vi "LVClass_ModalCoef ctor from copy.vi"(0 "ModalCoef (const)":refnum<class "ModalCoef.lvclass">, 5 "ModalCoef to copy":refnum<class "ModalCoef.lvclass">, 11 "error in (no error)":errorcluster) -> (4 "ModalCoef (new)":refnum<class "ModalCoef.lvclass">, 6 "ModalCoef to copy (dup)":refnum<class "ModalCoef.lvclass">, 15 "error out":errorcluster)   [LabVIEW 2020, in "ModalCoef.lvclass"]
doc: "ModalCoef constructor.\n\n--------------------------------------------------------------------------------\n\n<B>ModalCoefIn </B> : Constant Pointer to ModalCoef object.\n<B>ModalCoefOut </B> : Constant Pointer to ModalCoef object.\n<B>TypePhase </B> : TypePhase Phase mode reconstruction.\n<B>ErrorIn </B> : Error\n<B>ErrorOut </B> : Error\n\n--------------------------------------------------------------------------------"
uses:
  ModalCoef.lvclass
  Controls/Handle creation.ctl
  ModalCoef.lvclass/ModalCoef.ctl
  LVClass_ModalCoef Read ModalCoef.vi
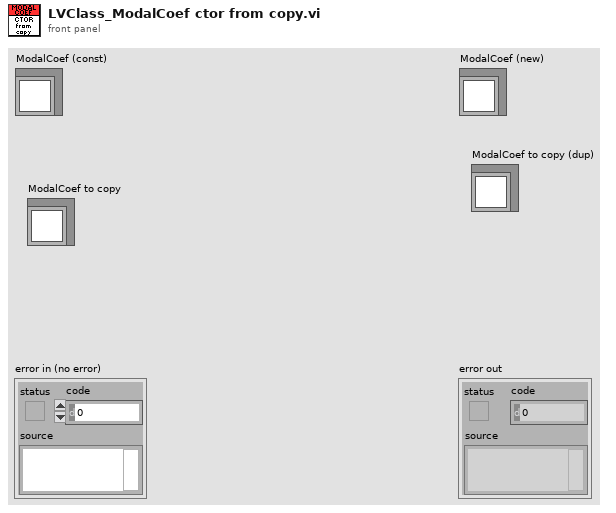
[diagram p1: front panel]
types:
  T1 = typedef "Handle creation.ctl" = enum16{"By ctor", "By write function"}
  T2 = typedef "ClassID.ctl" = i64
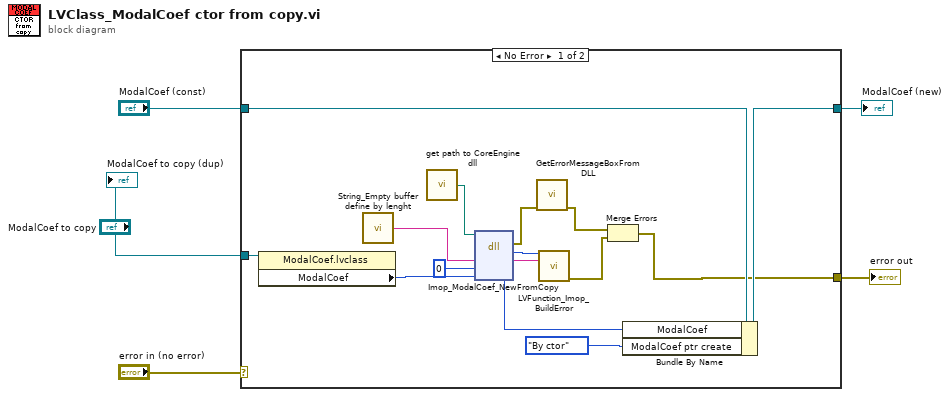
[diagram p0: block diagram]
diagram:
  n1 = case shown="No Error" "error in (no error)" {
    selector: "error in (no error)" -> [_ w22]
    tunnel: [w8 w22] -> w4
    tunnel: [w11 w21] -> w2
    tunnel: "ModalCoef (const)" -> [w12 w21]
    tunnel: "ModalCoef to copy" -> [w7 _]
    frame No Error {
      n2 = property class="ModalCoef.lvclass"(reference=w7) -> ("ModalCoef"=w6:T2)  [unwired: 1 in, 2 out]
      n3 = call "String_Empty buffer define by lenght.vi"() -> ("Empty buffer"=w20:string)  [unwired: 1 in]
      n4 = call "get path to CoreEngine dll.vi"() -> ("path to wavekit library"=w17:path)  [unwired: 14 in, 1 out]
      n5 = dll-call lib="D:/soft/HASO_v3/SVN_trunk/ImOpCoreEngine4_LV2011/DLLs/c_interface_vc100.dll" fn="Imop_ModalCoef_NewFromCopy"(path in=w17, "message"=w20, "ModalCoef"=0 ("Pupil"), "ModalCoefToCopy"=w6) -> (error out=w16:errorcluster, "return type"=w18:i32, "message"=w19:string, "ModalCoef"=w14:i64)  [unwired: 3 in, 1 out]
      n6 = call "GetErrorMessageBoxFromDLL.vi"("error IN"=w16) -> ("error OUT"=w10:errorcluster)  [unwired: 10 in]
      n7 = call "LVFunction_Imop_BuildError.vi"("code"=w18, "String to Prepend to source (\"\")"=w19) -> ("error out"=w9:errorcluster)  [unwired: 13 in]
      n8 = Merge Errors(w10, w9) -> (w8:errorcluster)
      n9 = Bundle By Name(cluster=w12, "ModalCoef"=w14, "ModalCoef ptr create"=Handle_creation."By ctor" ("Pupil ptr create")) -> (w11:refnum<class "ModalCoef.lvclass">)
    }
    frame Error {
    }
  }
  "error out" <- w4
  "ModalCoef (new)" <- w2
  "ModalCoef to copy (dup)" <- "ModalCoef to copy"
